vi "LJUD UE9RAW TimerCounter.vi"(5 "Comm Settings":T2={"Open LabJack "=TRUE, "Use USB"=TRUE, "IP Address"="192.168.1.209", "PortA"=52360, "PortB"=0}, 8 "error in (no error)":errorcluster, 10 "TimerCounter Config":T1={"TimerClockConfig"=0, "TimerClockDivisor"=1, "Do Enable/Disable"=FALSE, "Enable n Timers"=0, "Enable Counter0"=FALSE, "Enable Counter1"=FALSE, "UpdateReset Timers"=[FALSE, FALSE, FALSE, FALSE, FALSE, FALSE], "Reset Counter0"=FALSE, "Reset Counter1"=FALSE, "TimerModes"=[0, 0, 0, 0, 0, 0], "TimerValues"=[0, 0, 0, 0, 0, 0], "Counter0Mode"=0, "Counter1Mode"=0}, 11 "Handle In":i32) -> (0 "error out":errorcluster, 1 "Counter Reads":u32[](array[numeric]), 2 "Timer Reads":u32[](array[numeric]), 3 "Handle Out":i32)   [LabVIEW 2021]
panel:
  out "Read Array":u8[](array[numeric]) format="%.0x"
  out "Write Array":u8[](array[numeric])=[139, 242, 0, 160, 247, 0] format="%.0x"
  # "Timer0"
  # "Timer1"
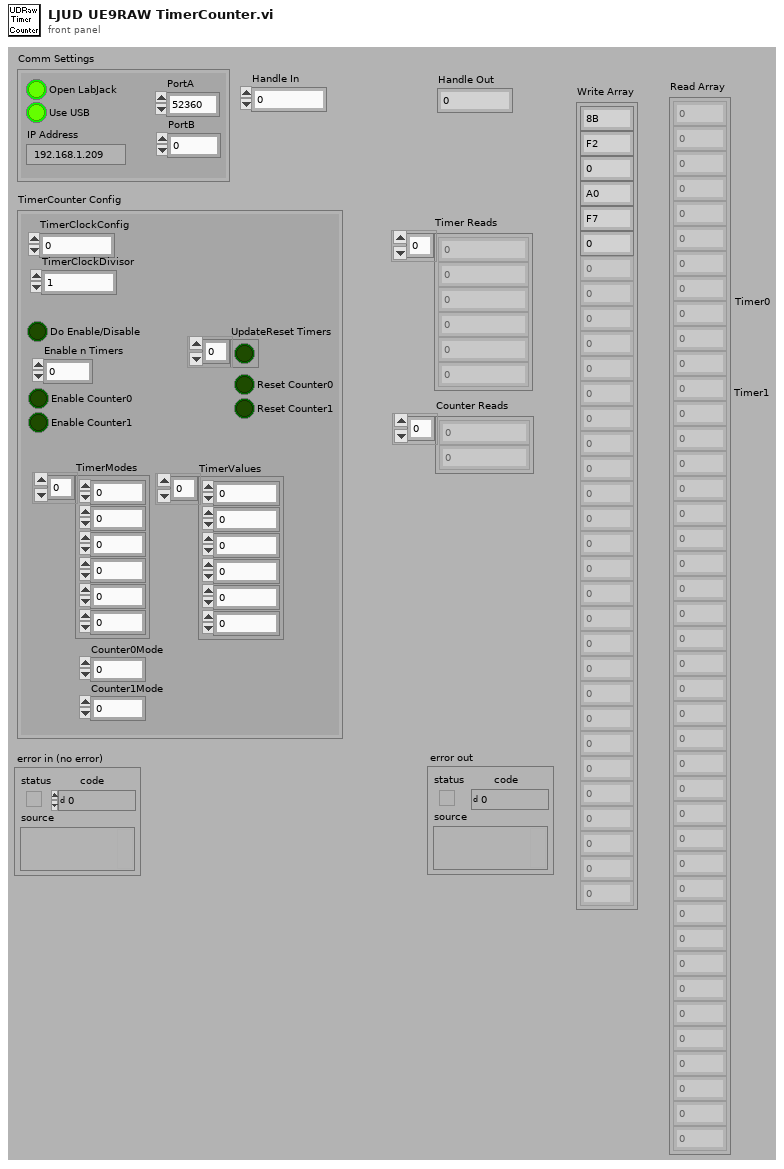
[diagram p1: front panel]
types:
  T1 = cluster{"TimerClockConfig":u8, "TimerClockDivisor":u8, "Do Enable/Disable":bool, "Enable n Timers":u8, "Enable Counter0":bool, "Enable Counter1":bool, "UpdateReset Timers":bool[], "Reset Counter0":bool, "Reset Counter1":bool, "TimerModes":u8[], "TimerValues":u16[], "Counter0Mode":u8, "Counter1Mode":u8}
  T2 = cluster{"Open LabJack ":bool, "Use USB":bool, "IP Address":string, "PortA":u16, "PortB":u16}
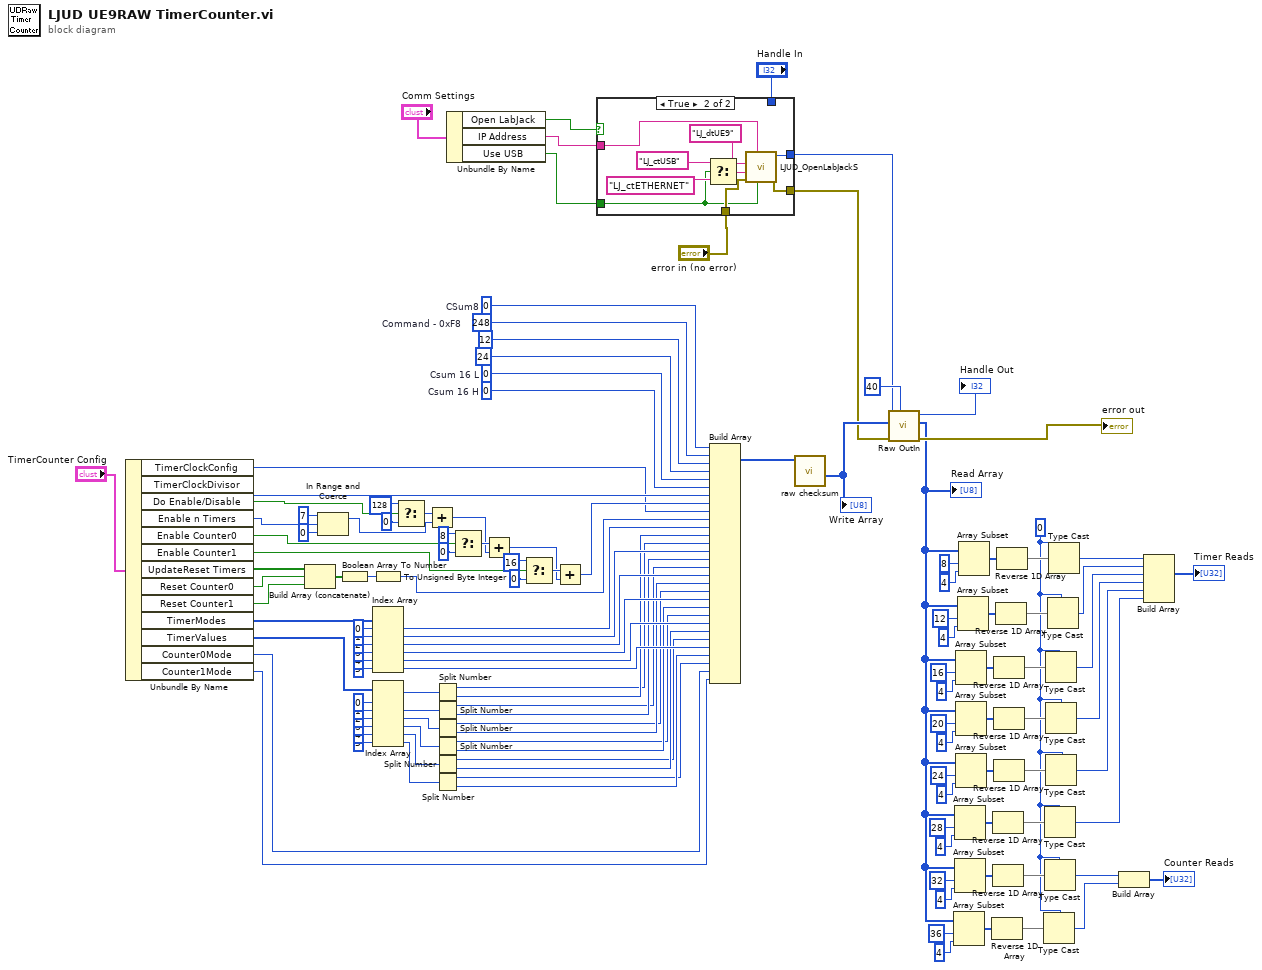
[diagram p0: block diagram]
diagram:
  w20 = u32 0
  w125 = u8 0  # Csum 16 H
  w126 = u8 0  # Csum 16 L
  w129 = u8 0  # CSum8
  w131 = u8 248  # Command - 0xF8
  n1 = Unbundle By Name("TimerCounter Config") -> ("TimerClockConfig"=w100:u8, "TimerClockDivisor"=w118:u8, "Do Enable/Disable"=w114:bool, "Enable n Timers"=w117:u8, "Enable Counter0"=w103:bool, "Enable Counter1"=w102:bool, "UpdateReset Timers"=w99:bool[], "Reset Counter0"=w98:bool, "Reset Counter1"=w97:bool, "TimerModes"=w93:u8[], "TimerValues"=w92:u16[], "Counter0Mode"=w79:u8, "Counter1Mode"=w78:u8)
  n2 = Build Array (concatenate)(w99, w98, w97) -> (w96:bool[])
  n3 = In Range and Coerce(upper limit=u8 7, x=w117, lower limit=u8 0) -> (coerced(x)=w111:u8)  [unwired: 1 out]
  n4 = Boolean Array To Number(Boolean array=w96) -> (number=w95:u32)
  n5 = To Unsigned Byte Integer(number=w95) -> (unsigned 8bit integer=w94:u8)
  n6 = Index Array(array=w93, index #1=0 ("Index"), index #2=1 ("Index"), index #3=2 ("Index"), index #4=3 ("Index"), index #5=4 ("Index"), index #6=5 ("Index")) -> (element #1=w77:u8, element #2=w76:u8, element #3=w75:u8, element #4=w74:u8, element #5=w73:u8, element #6=w72:u8)
  n7 = Index Array(array=w92, index #1=0 ("Index"), index #2=1 ("Index"), index #3=2 ("Index"), index #4=3 ("Index"), index #5=4 ("Index"), index #6=5 ("Index")) -> (element #1=w71:u16, element #2=w70:u16, element #3=w69:u16, element #4=w68:u16, element #5=w67:u16, element #6=w66:u16)
  n8 = Select(t=u8 128 ("upper limit"), s=w114, f=u8 0 ("upper limit")) -> (s? t:f=w110:u8)
  n9 = Add(x=w110, y=w111) -> (x+y=w105:u8)
  n10 = Split Number(x=w71) -> (hi(x)=w64:u8, lo(x)=w65:u8)
  n11 = Split Number(x=w70) -> (hi(x)=w62:u8, lo(x)=w63:u8)
  n12 = Split Number(x=w69) -> (hi(x)=w60:u8, lo(x)=w61:u8)
  n13 = Split Number(x=w68) -> (hi(x)=w58:u8, lo(x)=w59:u8)
  n14 = Split Number(x=w67) -> (hi(x)=w56:u8, lo(x)=w57:u8)
  n15 = Split Number(x=w66) -> (hi(x)=w54:u8, lo(x)=w55:u8)
  n16 = Unbundle By Name("Comm Settings") -> ("Open LabJack"=w3:bool, "IP Address"=w2:string, "Use USB"=w1:bool)
  n17 = Select(t=u8 8 ("upper limit"), s=w103, f=u8 0 ("upper limit")) -> (s? t:f=w109:u8)
  n18 = Add(x=w109, y=w105) -> (x+y=w104:u8)
  n19 = Select(t=u8 16 ("upper limit"), s=w102, f=u8 0 ("upper limit")) -> (s? t:f=w106:u8)
  n20 = Add(x=w106, y=w104) -> (x+y=w101:u8)
  n21 = case shown="True" w3 {
    tunnel: w2 -> [_ w136]
    tunnel: "error in (no error)" -> [w133 w140]
    tunnel: [w133 w139] -> w6
    tunnel: [w132 w137] -> w7
    tunnel: w1 -> [_ w138]
    tunnel: "Handle In" -> [w132 _]
    frame False {
    }
    frame True {
      n22 = Select(t="LJ_ctUSB" ("ConnectionType"), s=w138, f="LJ_ctETHERNET" ("ConnectionType")) -> (s? t:f=w134:string)
      n23 = call "LJUD_OpenLabJackS.vi"("FirstFound"=w138, "Address"=w136, "error in"=w140, "ConnectionType"=w134, "DeviceType"="LJ_dtUE9") -> ("error out"=w139:errorcluster, "Handle"=w137:i32)  [unwired: 4 in, 1 out]
    }
  }
  n24 = Build Array(w129, w131, u8 12 ("0x0E"), u8 24 ("0x00"), w126, w125, w118, w101, w100, w94, w77, w65, w64, w76, w63, w62, w75, w61, w60, w74, w59, w58, w73, w57, w56, w72, w55, w54, w79, w78) -> (w130:u8[])
  n25 = call "raw checksum.vi"("Array"=w130) -> ("Array Output"=w123:u8[])  [unwired: 3 in, 7 out]
  "Write Array" <- w123
  n26 = call "Raw OutIn.vi"("# of bytes to read in"=40 ("# of bytes to read"), "error in"=w6, "Raw Out"=w123, "Handle In"=w7) -> ("error out"=→"error out":errorcluster, "Raw In"=w21:u8[], "Handle Out"=→"Handle Out":i32)  [unwired: 4 in, 1 out]
  "Read Array" <- w21
  n27 = Array Subset(array=w21, index=36 ("Array Index"), length=4 ("Array Length")) -> (w25:u8[])
  n28 = Array Subset(array=w21, index=28 ("Array Index"), length=4 ("Array Length")) -> (w34:u8[])
  n29 = Array Subset(array=w21, index=32 ("Array Index"), length=4 ("Array Length")) -> (w26:u8[])
  n30 = Array Subset(array=w21, index=16 ("Array Index"), length=4 ("Array Length")) -> (w42:u8[])
  n31 = Array Subset(array=w21, index=20 ("Array Index"), length=4 ("Array Length")) -> (w30:u8[])
  n32 = Array Subset(array=w21, index=24 ("Array Index"), length=4 ("Array Length")) -> (w35:u8[])
  n33 = Array Subset(array=w21, index=12 ("Array Index"), length=4 ("Array Length")) -> (w49:u8[])
  n34 = Array Subset(array=w21, index=8 ("Array Index"), length=4 ("Array Length")) -> (w50:u8[])
  n35 = Reverse 1D Array(array=w25) -> (reversed array=w24:u8[])
  n36 = Reverse 1D Array(array=w34) -> (reversed array=w33:u8[])
  n37 = Reverse 1D Array(array=w26) -> (reversed array=w27:u8[])
  n38 = Reverse 1D Array(array=w42) -> (reversed array=w43:u8[])
  n39 = Reverse 1D Array(array=w30) -> (reversed array=w41:u8[])
  n40 = Reverse 1D Array(array=w35) -> (reversed array=w36:u8[])
  n41 = Reverse 1D Array(array=w49) -> (reversed array=w48:u8[])
  n42 = Reverse 1D Array(array=w50) -> (reversed array=w51:u8[])
  n43 = Type Cast(type=w20, x=w24) -> (*(type *) &x=w11:u32)
  n44 = Type Cast(type=w20, x=w33) -> (*(type *) &x=w13:u32)
  n45 = Type Cast(type=w20, x=w27) -> (*(type *) &x=w12:u32)
  n46 = Type Cast(type=w20, x=w43) -> (*(type *) &x=w16:u32)
  n47 = Type Cast(type=w20, x=w41) -> (*(type *) &x=w15:u32)
  n48 = Type Cast(type=w20, x=w36) -> (*(type *) &x=w14:u32)
  n49 = Type Cast(type=w20, x=w48) -> (*(type *) &x=w17:u32)
  n50 = Type Cast(type=w20, x=w51) -> (*(type *) &x=w19:u32)
  n51 = Build Array(w12, w11) -> (→"Counter Reads":u32[])
  n52 = Build Array(w19, w17, w16, w15, w14, w13) -> (→"Timer Reads":u32[])
